vi "Actor Core.vi"(8 "error in":errorcluster, 11 "Sim User Console Actor in":refnum<class "Sim User Console Actor.lvclass">) -> (0 "error out":errorcluster, 3 "Actor out":refnum<class "Actor.lvclass">)   [LabVIEW 2022 SP3, in "Sim User Console Actor.lvlib" / "Sim User Console Actor.lvclass"]
doc: "(<B>Filename</B>: Actor Framework.lvlib:Actor.lvclass:Actor Core.vi)\n\nReceives messages to the actor, reacts to them, and initiates any error handling that may shut the actor down.\n\nDescendant classes may override this VI to append parallel tasks for the actor to complete while it handles messages. Overrides use the Call Parent Class Method node."
uses:
  Sim User Console Actor.lvclass
  Sim User Console Actor.lvclass/Sim User Console Actor.ctl
  <vilib>/ActorFramework/Stop Msg/Stop Msg.lvclass
  <vilib>/ActorFramework/Actor/Actor.lvclass
  Abstract User Console Actor/Abstract User Console Actor/Abstract User Console Actor.lvclass
  C:/Workspace/CLA/Elevator AF_2022/Abstract User Console Actor/Abstract User Console Actor/Abstract User Console Actor.lvclass
  C:/Program Files/National Instruments/LabVIEW 2022/vi.lib/ActorFramework/Actor/Actor.lvclass
  C:/Workspace/CLA/Elevator AF_2022/Sim User Console Actor/Abstract User Console Actor/Sim User Console Actor.lvclass
  Abstract User Console Actor/Abstract User Console Actor/Door Buttons.ctl
  Abstract User Console Actor/Abstract User Console Actor/Elevator Call.ctl
  Abstract User Console Actor/Abstract User Console Actor/Floor Selection.ctl
panel:
  in  "Emergency":bool
  in  "Floor Selection":T1
  in  "Elevator Call":T2
  in  "Door Buttons":T3
  # "[Covers: UI2]\n[Covers: UI2A] \n[Covers: UI2A1] \n[Covers: UI2A2]"
  # "[Covers: UI2B] \n[Covers: UI2B1] \n[Covers: UI2B2]"
  # "[Covers: UI2C] \n[Covers: UI2C1] \n[Covers: UI2C2] \n[Covers: UI2C3]"
  # "[Covers: UI2D] \n[Covers: UI2D1]"
  # "[Covers: UI1]"
  # "Fourth Floor"
  # "Third Floor"
  # "Second Floor"
  # "First Floor"
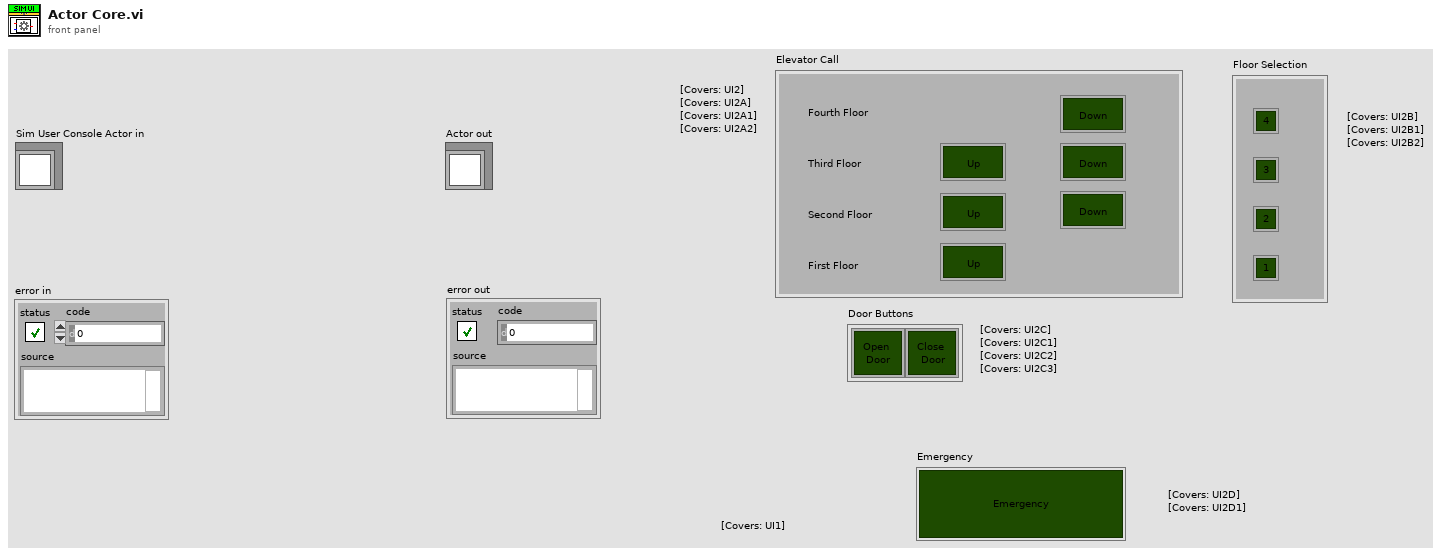
[diagram p1: front panel]
types:
  T1 = typedef "Abstract User Console Actor.lvlib/Abstract User Console Actor.lvclass/Floor Selection.ctl" = cluster{"Floor4":bool, "Floor 3":bool, "Floor2":bool, "Floor1":bool}
  T2 = typedef "Abstract User Console Actor.lvlib/Abstract User Console Actor.lvclass/Elevator Call.ctl" = cluster{"Up":bool, "Up 2":bool, "Up 3":bool, "Down":bool, "Down 2":bool, "Down 3":bool}
  T3 = typedef "Abstract User Console Actor.lvlib/Abstract User Console Actor.lvclass/Door Buttons.ctl" = cluster{"Open Door":bool, "Close Door":bool}
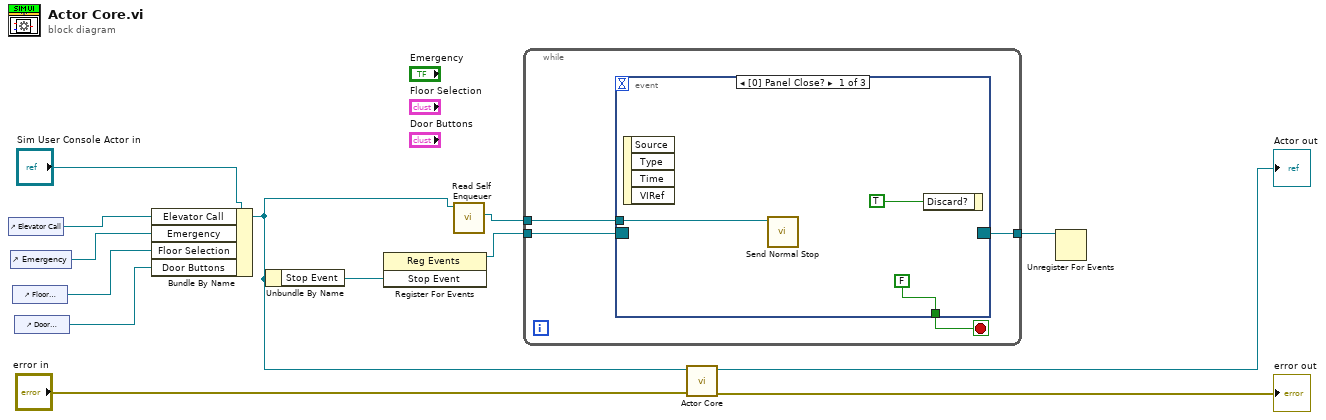
[diagram p0: block diagram]
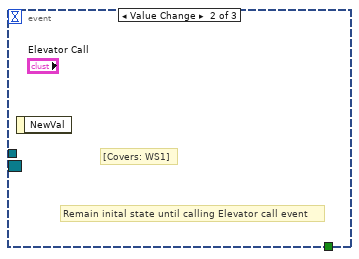
[diagram p2: hidden frame]
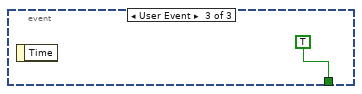
[diagram p3: hidden frame]
diagram:
  n1 = control-ref of="Elevator Call"() -> (w8:refnum<vi>)
  n2 = control-ref of="Emergency"() -> (w7:refnum<vi>)
  n3 = control-ref of="Floor Selection"() -> (w6:refnum<vi>)
  n4 = control-ref of="Door Buttons"() -> (w5:refnum<vi>)
  n5 = Bundle By Name(cluster="Sim User Console Actor in", "Elevator Call"=w8, "Emergency"=w7, "Floor Selection"=w6, "Door Buttons"=w5) -> (w4:refnum<class "Sim User Console Actor.lvclass">)
  n6 = Unbundle By Name(w4) -> ("Stop Event"=w3:refnum<user-event>)
  n7 = register-events(w3) -> (reference out=w2:refnum<event-registration>)  [unwired: 2 in, 1 out]
  n8 = call <vilib>:"Read Self Enqueuer.vi"("Actor"=w4) -> ("Self Enqueuer"=w10:refnum<class "Message Enqueuer.lvclass">)  [unwired: 10 in]
  n9 = while {
    tunnel: w10 -> [w16]
    tunnel: w2 -> [w15]
    tunnel: [w14] -> w1
    stop <- w17 stop-if-true
    n10 = event shown="[0] Panel Close?" {
      selector: w15 -> [_ _ _]
      dyn-events: [_ _ _] -> w14
      timeout: _ -> [_ _ _]
      tunnel: [FALSE _ TRUE] -> w17
      tunnel: w16 -> [w19 _ _]
      event Panel Close? {
        n11 = event-data() -> ()  [unwired: 1 in, 4 out]
        n12 = call <vilib>:"Send Normal Stop.vi"("Message Enqueuer"=w19) -> ()  [unwired: 10 in, 1 out]
        n13 = event-data("Discard?"=TRUE) -> ()  [unwired: 1 in, 1 out]
      }
      event Value Change {
        # "Remain inital state until calling Elevator call event"
        # "[Covers: WS1]"
        n14 = event-data() -> ()  [unwired: 1 in, 1 out]
      }
      event User Event {
        n15 = event-data() -> ()  [unwired: 1 in, 1 out]
      }
    }
  }
  n16 = call-parent "Actor Core.vi"("error in"="error in", "Actor in"=w4) -> ("error out"=→"error out":errorcluster, "Actor out"=→"Actor out":refnum<class "Actor.lvclass">)  [unwired: 8 in]
  n17 = Unregister For Events(event registration refnum=w1) -> ()  [unwired: 1 in, 1 out]
